vi "main.vi"() -> ()   [LabVIEW 2019]
uses:
  <vilib>/httpClient/LabVIEWHTTPClient.lvlib
panel:
  out "Cartesian coordinates":cluster{"x":string, "y":string, "z":string}
  out "Rotational components":cluster{"rx":string, "ry":string, "rz":string}
  out "Joint positions":T1
  in  "Parameters":dbl[](array[numeric])
  in  "Method names":string(combo)
  in  "URL":string="10.42.0.1:8080/xml-rpc"
  in  "password":string="WZA3P9"
  in  "username":string="WZA3P9"
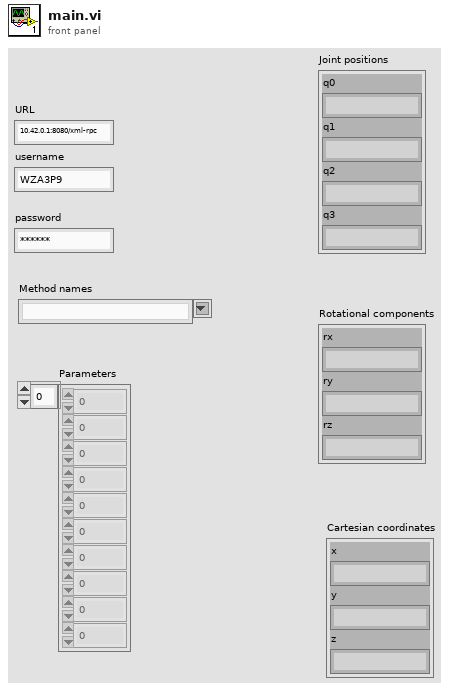
[diagram p1: front panel]
types:
  T1 = cluster{"q0":string, "q1":string, "q2":string, "q3":string}
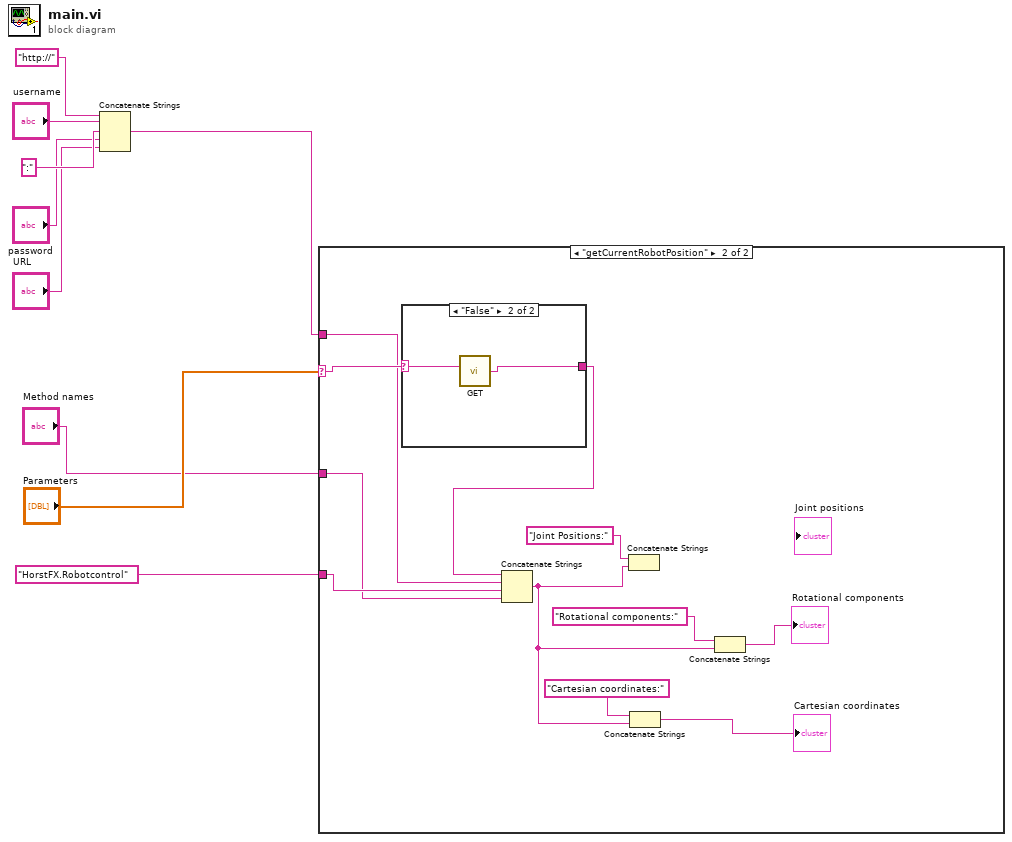
[diagram p0: block diagram]
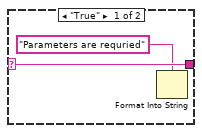
[diagram p3: hidden frame]
diagram:
  n1 = Concatenate Strings("http://", "username", ":", "password", "URL") -> (w3:string)
  n2 = case shown="\"getCurrentRobotPosition\"" "Parameters" {
    selector: "Parameters" -> [_ w20]
    tunnel: w3 -> [_ w13]
    tunnel: "HorstFX.Robotcontrol" -> [_ w12]
    tunnel: "Method names" -> [_ w11]
    frame "False", Default {
    }
    frame "getCurrentRobotPosition" {
      n3 = case shown="\"False\"" w20 {
        selector: w20 -> [w22 w24]
        tunnel: [w22 w23] -> w10
        frame "True" {
          n4 = Format Into String(format string="Parameters are requried") -> ()  [unwired: 3 in, 2 out]
        }
        frame "False" {
          n5 = call <vilib>:"GET.vi"("url"=w24) -> ("body"=w23:string)  [unwired: 11 in, 3 out]
        }
      }
      n6 = Concatenate Strings(w10, w13, w12, w11) -> (w17:string)
      n7 = Concatenate Strings("Joint Positions:", w17) -> ()  [unwired: 1 out]
      n8 = Concatenate Strings("Cartesian coordinates:", w17) -> (→"Cartesian coordinates":string)
      n9 = Concatenate Strings("Rotational components:", w17) -> (→"Rotational components":string)
    }
  }
